vi "Measure Voltage.vi"(8 "error in (no error)":errorcluster, 10 "Output":T1, 11 "VISA resource name":refnum<visa-resource-name>) -> (0 "error out":errorcluster, 1 "measured V":dbl, 2 "Output":T1, 3 "VISA Refnum out":refnum<visa-resource-name>)   [LabVIEW 2019, in "RP100.lvlib"]
uses:
  RP100.lvlib
  Inst.RP100/Typedefs/Channel--Num.ctl
  Inst.RP100/Inst.RP100.lvclass
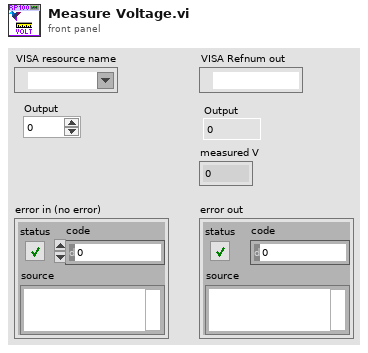
[diagram p1: front panel]
types:
  T1 = typedef "Inst.RP100.lvlib/Inst.RP100.lvclass/Channel--Num.ctl" = i32
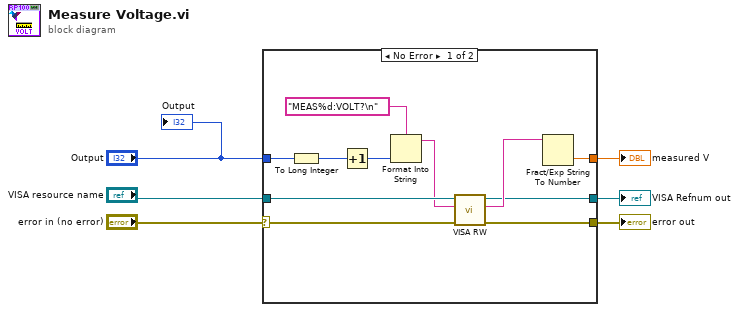
[diagram p0: block diagram]
diagram:
  n1 = case shown="No Error" "error in (no error)" {
    selector: "error in (no error)" -> [w14 w19]
    tunnel: [w10 w18] -> w6
    tunnel: [w9 w19] -> w5
    tunnel: [w17 _] -> w4
    tunnel: "VISA resource name" -> [w13 w18]
    tunnel: "Output" -> [w16 _]
    frame No Error {
      n2 = To Long Integer(number=w16) -> (32bit integer=w8:T1)
      n3 = Increment(x=w8) -> (x+1=w7:T1)
      n4 = Format Into String(format string="MEAS%d:VOLT?\n", w7) -> (resulting string=w12:string)  [unwired: 2 in, 1 out]
      n5 = call "VISA RW.vi"("error in (no error)"=w14, "Write"=w12, "VISA Refnum in"=w13) -> ("error out"=w9:errorcluster, "Read"=w11:string, "VISA Refnum out"=w10:refnum<visa-resource-name>)  [unwired: 6 in]
      n6 = Fract/Exp String To Number(string=w11) -> (number=w17:dbl)  [unwired: 3 in, 1 out]
    }
    frame Error {
    }
  }
  "measured V" <- w4
  "VISA Refnum out" <- w6
  "error out" <- w5
  "Output" <- "Output"
